vi "Check System Definition for Channel Dependency.vi"() -> ()   [LabVIEW 2025]
uses:
  Controls/Replacement Channels.ctl
  NationalInstruments.VeriStand.SystemDefinitionAPI
panel:
  in  "Replacement Channels":T1={"Channel to Replace"="Targets/Controller/User Channels/User Channel 2", "Replacement Channel"="Targets/Controller/User Channels/User Channel 1"}
  out "Replacement Log":string[](array[string])
  in  "System Definition File Path":path=path "C:/dev/VCOM-SysDef-Utility/VCOM Config System Definition Utility/VeriStand Example Project/Example Project/Example Project.nivssdf"
  out "error out":errorcluster
  in  "error in (no error)":errorcluster
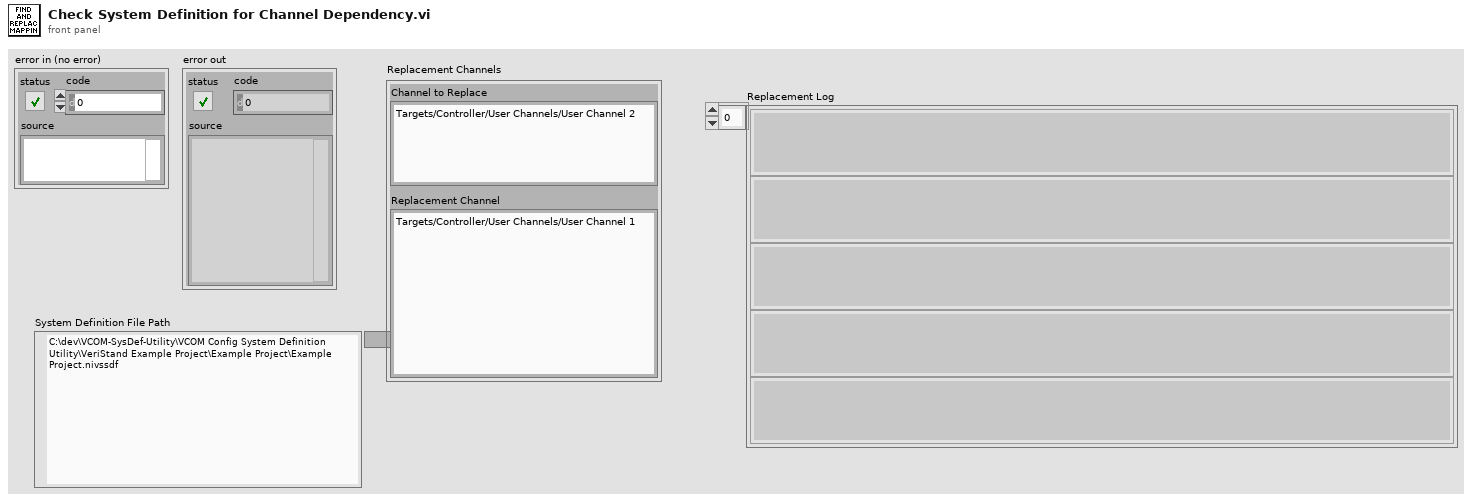
[diagram p1: front panel]
types:
  T1 = typedef "Replacement Channels.ctl" = cluster{"Channel to Replace":string, "Replacement Channel":string}
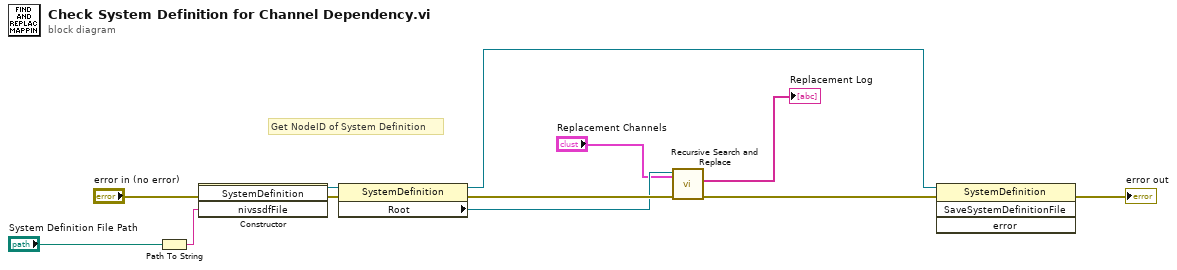
[diagram p0: block diagram]
diagram:
  # "Get NodeID of System Definition"
  n1 = Path To String(path="System Definition File Path") -> (string=w12:string)
  n2 = constructor class="SystemDefinition"(error in="error in (no error)", "nivssdfFile"=w12) -> (reference out=w10:refnum<k24>, error out=w11:errorcluster)  [unwired: 2 in, 2 out]
  n3 = property class="SystemDefinition"(reference=w10, error in=w11) -> (reference out=w4:refnum<k24>, error out=w7:errorcluster, "Root"=w6:refnum<k24>)
  n4 = call "Recursive Search and Replace.vi"("Replacement Channels"="Replacement Channels", "error in (no error)"=w7, ".NET Refnum"=w6) -> ("error out"=w3:errorcluster, "Replacement Log"=→"Replacement Log":string[])  [unwired: 7 in]
  n5 = invoke class="SystemDefinition" method="SaveSystemDefinitionFile"(reference=w4, error in=w3) -> (error out=→"error out":errorcluster)  [unwired: 2 in, 3 out]
